vi "Distributor - Launch Actors.vi"(8 "error in (no error)":errorcluster, 11 "Parent_Class in":refnum<class "Message_Distributor_Class.lvclass">) -> (0 "error out":errorcluster, 3 "Parent_Class out":refnum<class "Message_Distributor_Class.lvclass">)   [LabVIEW 2023, in "Actor_Message_Distributor.lvlib" / "Message_Distributor_Class.lvclass"]
uses:
  Message_Distributor_Class.lvclass
  C:/Program Files/National Instruments/LabVIEW 2023/vi.lib/ActorFramework/Actor/Actor.lvclass
  GUI/GUI_Class.lvclass
  C:/Users/rodri/LabVIEW_Labs/LabVIEW_GitHub/LV_AF_Project/AF_Architecture/Abstraction_Interface_Class/Abstraction_Interface_Class.lvclass
  Console/Console_Class.lvclass
  SW_Interface/SW_Interface_Class.lvclass
  Logging/Logging_Class.lvclass
  Error_Engine/Error_Emgime_Class.lvclass
  Embedded_DB/Embedded_DB_Class.lvclass
  Console/Console_Class.lvclass/Console_Class.ctl
  GUI/GUI_Class.lvclass/GUI_Class.ctl
  <vilib>/ActorFramework/Actor/Actor.lvclass/Actor.ctl
  <vilib>/ActorFramework/Message Enqueuer/Message Enqueuer.lvclass/Message Enqueuer.ctl
  Message_Distributor_Class.lvclass/Message_Distributor_Class.ctl
  <vilib>/Utility/error.llb/Trim Whitespace.vi
  <vilib>/ActorFramework/Message Enqueuer/Init from Existing Queue.vi
  <vilib>/Utility/error.llb/Trim Whitespace One-Sided.vi
  Abstraction_Interface_Class/Abstraction_Interface_Class.lvclass
  <vilib>/Utility/LVClass/Get LV Class Name.vi
  <vilib>/ActorFramework/Message Enqueuer/Message Enqueuer.lvclass
  <vilib>/ActorFramework/Actor/Actor.lvclass
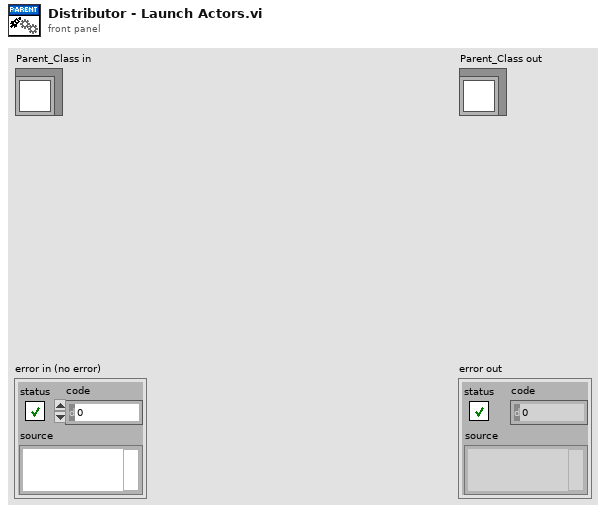
[diagram p1: front panel]
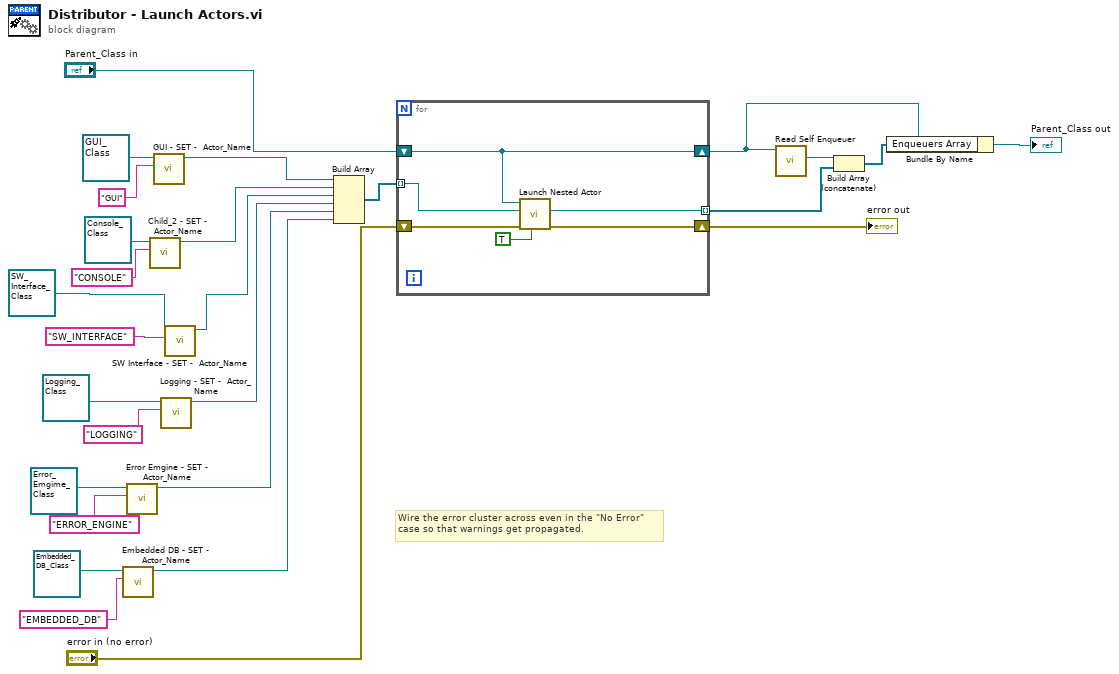
[diagram p0: block diagram]
diagram:
  # "Wire the error cluster across even in the \"No Error\"\ncase so that warnings get propagated."
  n1 = call "Embedded DB - SET - Actor_Name.vi"("Actor_Name IN"="EMBEDDED_DB", "Child_6_Class in"=refnum<class "Embedded_DB_Class.lvclass"> refnum ("Embedded_DB_Actor.lvlib:Embedded_DB_Class.lvclass")) -> ("Child_6_Class out"=w1:refnum<class "Embedded_DB_Class.lvclass">)  [unwired: 7 in, 2 out]
  n2 = call "Error Emgine - SET - Actor_Name.vi"("Actor_Name IN"="ERROR_ENGINE", "Child_5_Class in"=refnum<class "Error_Emgime_Class.lvclass"> refnum ("Error_Engine_Actor.lvlib:Error_Emgime_Class.lvclass")) -> ("Child_5_Class out"=w2:refnum<class "Error_Emgime_Class.lvclass">)  [unwired: 7 in, 2 out]
  n3 = call "Child_2 - SET -  Actor_Name.vi"("Actor_Name"="CONSOLE", "Child_2_Class in"=refnum<class "Console_Class.lvclass"> refnum ("Actor_Child_2.lvlib:Child_2_Class.lvclass")) -> ("Child_2_Class out"=w13:refnum<class "Console_Class.lvclass">)  [unwired: 7 in, 2 out]
  n4 = call "GUI - SET -  Actor_Name.vi"("Actor_Name"="GUI", "Child_1_Class in"=refnum<class "GUI_Class.lvclass"> refnum ("Actor_Child_1.lvlib:Child_1_Class.lvclass")) -> ("Child_1_Class out"=w14:refnum<class "GUI_Class.lvclass">)  [unwired: 8 in, 1 out]
  n5 = call "Logging - SET -  Actor_Name.vi"("Actor_Name IN"="LOGGING", "Logging_Class in"=refnum<class "Logging_Class.lvclass"> refnum ("Logging.lvlib:Logging_Class.lvclass")) -> ("Logging_Class out"=w7:refnum<class "Logging_Class.lvclass">)  [unwired: 7 in, 2 out]
  n6 = call "SW Interface - SET -  Actor_Name.vi"("Actor_Name"="SW_INTERFACE", "SW_Interface_Actor.lvlib:SW_Interface_Class.lvclass"=refnum<class "SW_Interface_Class.lvclass"> refnum) -> ("SW_Interface_Actor.lvlib:SW_Interface_Class.lvclass 2"=w11:refnum<class "SW_Interface_Class.lvclass">)  [unwired: 7 in, 2 out]
  n7 = Build Array(w14, w13, w11, w7, w2, w1) -> (w27:refnum<class "Abstraction_Interface_Class.lvclass">[])
  n8 = for {
    tunnel: w27 -> [w31] mode=indexing
    shift-right: [w32] -> w24
    shift-left: "error in (no error)" -> [w33]
    shift-right: [w30] -> w21
    shift-left: "Parent_Class in" -> [w30]
    tunnel: [w28] -> w22 mode=indexing
    n9 = call <vilib>:"Launch Nested Actor.vi"("Open Actor Core front panel? (F)"=TRUE, "error in (no error)"=w33, "Nested Actor"=w31, "Caller Actor in"=w30) -> ("error out"=w32:errorcluster, "Nested Actor's Enqueuer"=w28:refnum<class "Message Enqueuer.lvclass">)  [unwired: 5 in, 1 out]
  }
  "error out" <- w24
  n10 = call <vilib>:"Read Self Enqueuer.vi"("Actor"=w21) -> ("Self Enqueuer"=w23:refnum<class "Message Enqueuer.lvclass">)  [unwired: 10 in]
  n11 = Build Array (concatenate)(w23, w22) -> (w20:refnum<class "Message Enqueuer.lvclass">[])
  n12 = Bundle By Name(cluster=w21, "Enqueuers Array"=w20) -> (→"Parent_Class out":refnum<class "Message_Distributor_Class.lvclass">)
